vi "Comma-separated-list extractor.vi"(5 "error in (no error)":errorcluster, 8 "In_list":string[](array[string])) -> (0 "error out":errorcluster, 3 "List_Out":string[](array[string]))   [LabVIEW 2014]
panel:
  out "strng":string
  out "Intmdt List":string[](array[string])
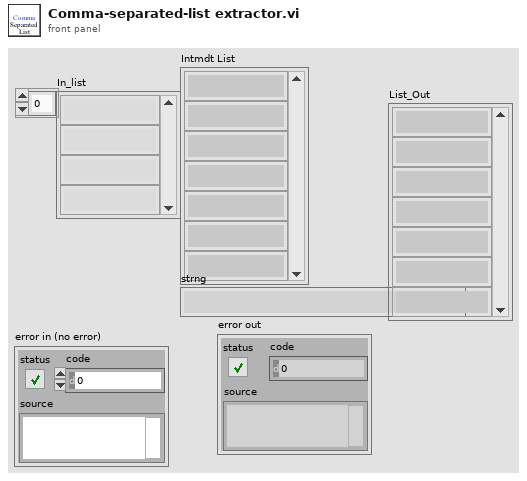
[diagram p1: front panel]
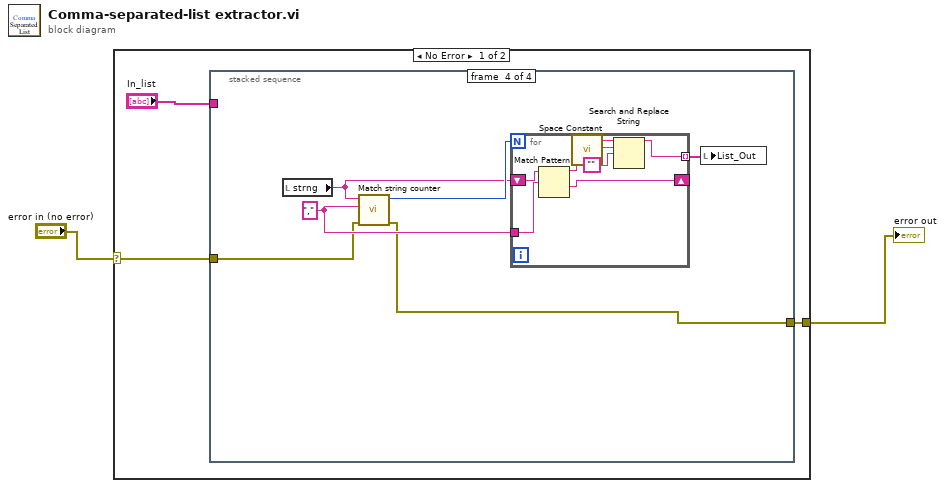
[diagram p0: block diagram]
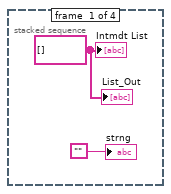
[diagram p2: hidden frame]
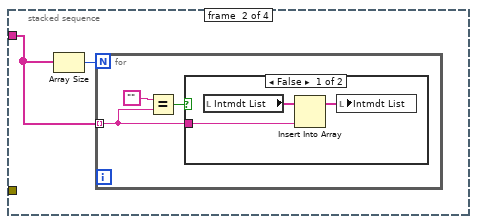
[diagram p3: hidden frame]
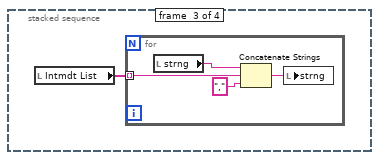
[diagram p5: hidden frame]
diagram:
  n1 = case shown="No Error" "error in (no error)" {
    selector: "error in (no error)" -> [w4 w34]
    tunnel: [w3 w34] -> w1
    frame No Error {
      n2 = stacked-sequence {
        tunnel: "In_list" -> [_ w8 _ _]
        tunnel: w4 -> [_ _ _ w23]
        tunnel: [_ _ _ w22] -> w3
        frame #0 {
          w7 = string[] [] ("Intmdt List")
          "Intmdt List" <- w7
          "List_Out" <- w7
          "strng" <- ""
        }
        frame #1 {
          n3 = Array Size(array=w8) -> (size(s)=w9:i32)
          n4 = for {
            N: w9 -> [_]
            tunnel: w8 -> [w10] mode=indexing
            n5 = Equal?(x="", y=w10) -> (x = y?=w11:bool)
            n6 = case shown="False" w11 {
              tunnel: w10 -> [w13 _]
              frame False {
                n7 = local read "Intmdt List"() -> (w14:string[])
                n8 = Insert Into Array(array=w14, new element=w13) -> (w15:string[])  [unwired: 1 in]
                n9 = local write "Intmdt List"(w15) -> ()
              }
              frame True {
              }
            }
          }
        }
        frame #2 {
          n10 = local read "Intmdt List"() -> (w16:string[])
          n11 = for {
            tunnel: w16 -> [w19] mode=indexing
            n12 = local read "strng"() -> (w20:string)
            n13 = Concatenate Strings(w20, w19, "," ("string")) -> (w18:string)
            n14 = local write "strng"(w18) -> ()
          }
        }
        frame #3 {
          w24 = "," ("Match String")
          n15 = local read "strng"() -> (w25:string)
          n16 = call "Match string counter.vi"("error in (no error)"=w23, "Match String"=w24, "Input string"=w25) -> ("error out"=w22:errorcluster, "Count"=w26:i32)  [unwired: 7 in]
          n17 = for {
            N: w26 -> [_]
            tunnel: w24 -> [w33]
            shift-right: [w32] -> _
            shift-left: w25 -> [w31]
            tunnel: [w27] -> w21 mode=indexing
            n18 = Match Pattern(string=w31, regular expression=w33) -> (before substring=w30:string, after substring=w32:string)  [unwired: 1 in, 2 out]
            n19 = call <vilib>:"Space Constant.vi"() -> ("String"=w29:string)
            n20 = Search and Replace String(input string=w30, search string=w29, replace string="") -> (result string=w27:string)  [unwired: 5 in, 3 out]
          }
          n21 = local write "List_Out"(w21) -> ()
        }
      }
    }
    frame Error {
    }
  }
  "error out" <- w1
